vi "Send DisplayResult_UI.vi"(7 "Message Priority (Normal)":T3=enum."Normal", 8 "error in (no error)":errorcluster, 10 "Result Cluster":T1, 11 "Message Enqueuer":refnum<class "Message Enqueuer.lvclass">) -> (0 "error out":errorcluster, 3 "Message Enqueuer out":refnum<class "Message Enqueuer.lvclass">)   [LabVIEW 2019, in "ZenGage v3.0 UI.lvlib" / "DisplayResult_UI Msg.lvclass"]
doc: "This VI sends the message to an actor."
uses:
  DisplayResult_UI Msg.lvclass
  <vilib>/ActorFramework/Message Enqueuer/Message Enqueuer.lvclass
  C:/Program Files/National Instruments/LabVIEW 2019/vi.lib/ActorFramework/Message/Message.lvclass
  <vilib>/ActorFramework/Message Enqueuer/Message Priority.ctl
  <vilib>/vision/Image Controls.llb/IMAQ Image.ctl
  User Interface Actor/Type Definitions/Inspection/Result Cluster.ctl
  User Interface Actor/ZenGage v3.0 UI.lvclass
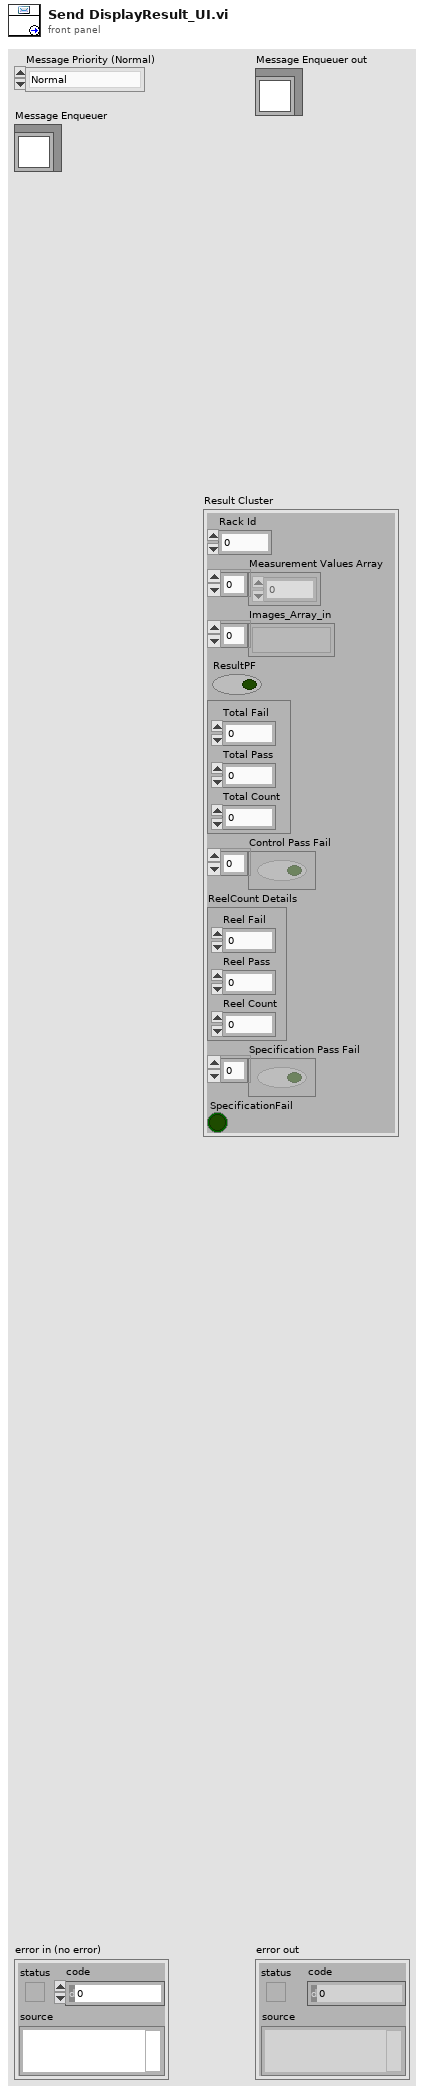
[diagram p1: front panel]
types:
  T1 = typedef "ZenGage v3.0 UI.lvclass/Result Cluster.ctl" = cluster{"Rack Id":u64, "Measurement Values Array ":dbl[], "Images_Array_in":T2[], "ResultPF":bool, "Production count details":cluster{"Total Count":dbl, "Total Pass":dbl, "Total Fail":dbl}, "Control Pass Fail":bool[], "ReelCount Details":cluster{"Reel Count":dbl, "Reel Pass":dbl, "Reel Fail":dbl}, "Specification Pass Fail":bool[], "SpecificationFail":bool}
  T2 = typedef "IMAQ Image.ctl" = refnum<image>
  T3 = typedef "Actor Framework.lvlib/Message Enqueuer.lvclass/Message Priority.ctl" = enum16{"Low", "Normal", "High"}
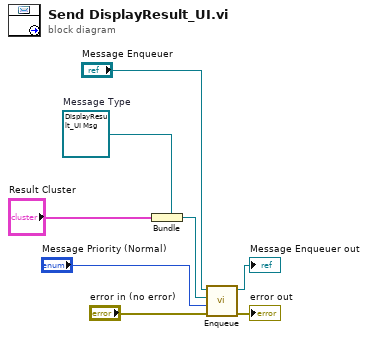
[diagram p0: block diagram]
diagram:
  w5 = refnum<class "DisplayResult_UI Msg.lvclass"> refnum  # Message Type
  n1 = Bundle(cluster=w5, "Result Cluster") -> (w4:refnum<class "DisplayResult_UI Msg.lvclass">)
  n2 = call <vilib>:"Enqueue.vi"("error in (no error)"="error in (no error)", "Message Priority (Normal)"="Message Priority (Normal)", "Message"=w4, "Message Enqueuer in"="Message Enqueuer") -> ("error out"=→"error out":errorcluster, "Message Enqueuer out"=→"Message Enqueuer out":refnum<class "Message Enqueuer.lvclass">)  [unwired: 6 in]
